vi "Get Package Dependencies from BuildSpec.vi"(0 "Path":path=path "C:/validation/Validation Framework/VI Packages/Build Specification/Validation Class/CLIVE.vipb", 11 "error in (no error)":errorcluster) -> (6 "Dependencies":string[](array[string])=["cirrus_ins_driver_silicon_delta >=2.0.0.1", "cirrus_ins_drivers_agilent_3631a >=2.0.0.1", "cirrus_ins_drivers_digital_interface >=2.1.0.1", "cirrus_ins_drivers_dmm_class >=2.0.0.1", "cirrus_ins_drivers_instek_psmx >=2.0.0.1", "cirrus_ins_drivers_ni_dc_power >=2.0.0.1", "cirrus_ins_drivers_ni_dmm >=2.0.0.1", "cirrus_ins_drivers_ni_scope >=2.0.0.1", "cirrus_ins_drivers_power_supply >=2.0.0.1", "cirrus_ins_drivers_tektronix_scope >=2.0.0.1", "ni_lib_amc >=3.3.1.22", "openg.org_lib_openg_toolkit >=4.0.1.9", "reusables >=1.3.0.2", "vigods_com_lib_advanced_encryption_standard_(aes) >=1.0.0.12"], 15 "error out":errorcluster)   [LabVIEW 2017, in "CL_G3_VIPMUtilities.lvlib"]
uses:
  CL_G3_VIPMUtilities.lvlib
  <vilib>/xml/Close Reference(Node).vi
  <vilib>/xml/Close Reference(NdList).vi
  <resource>/objmgr/DOMUserDefRef.rc
  <vilib>/xml/NI_XML.lvlib
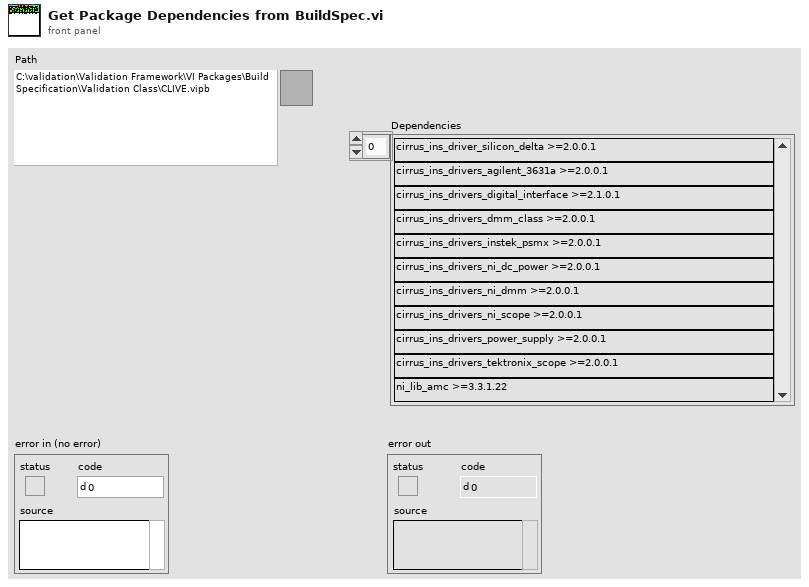
[diagram p1: front panel]
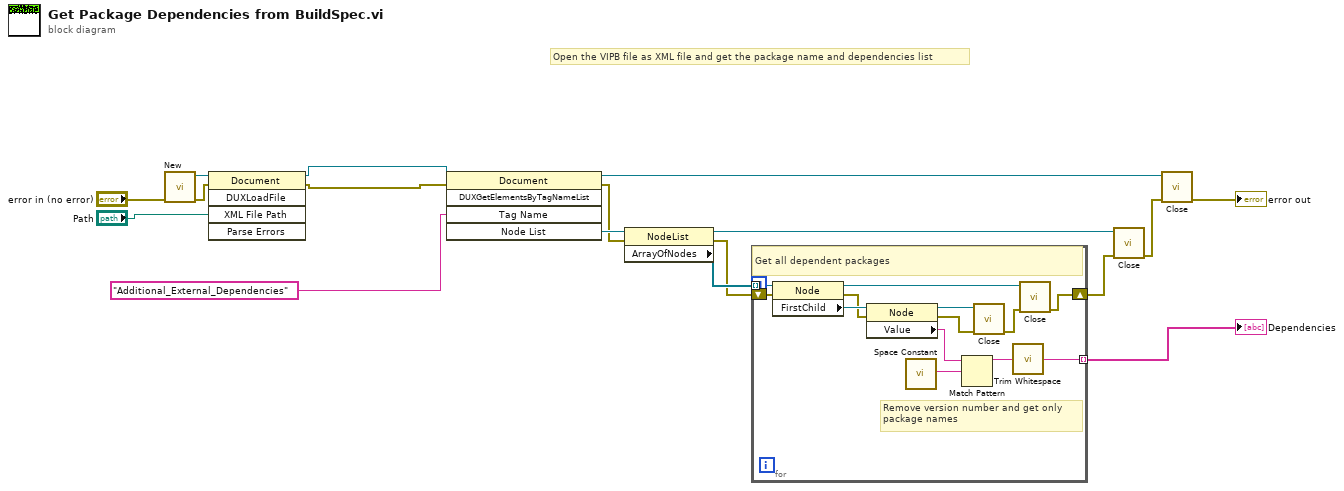
[diagram p0: block diagram]
diagram:
  # "Open the VIPB file as XML file and get the package name and dependencies list"
  n1 = call <vilib>:"New.vi"("error in (no error)"="error in (no error)") -> ("error out"=w16:errorcluster, "DOM document out"=w17:refnum<k20>)  [unwired: 7 in]
  n2 = invoke class="Document" method="DUXLoadFile"(reference=w17, error in=w16, "XML File Path"="Path") -> (reference out=w2:refnum<k20>, error out=w1:errorcluster)  [unwired: 2 in, 3 out]
  n3 = invoke class="Document" method="DUXGetElementsByTagNameList"(reference=w2, error in=w1, "Tag Name"="Additional_External_Dependencies") -> (reference out=w14:refnum<k20>, error out=w8:errorcluster, "Node List"=w13:refnum<k20>)  [unwired: 2 in, 2 out]
  n4 = property class="NodeList"(reference=w13, error in=w8) -> (reference out=w6:refnum<k20>, error out=w7:errorcluster, "ArrayOfNodes"=w9:refnum<k20>[])
  n5 = for {
    tunnel: [w18] -> w10 mode=indexing
    tunnel: w9 -> [w30] mode=indexing
    shift-right: [w22] -> w5
    shift-left: w7 -> [w28]
    # "Remove version number and get only\npackage names"
    # "Get all dependent packages"
    n6 = property class="Node"(reference=w30, error in=w28) -> (reference out=w24:refnum<k20>, error out=w25:errorcluster, "FirstChild"=w29:refnum<k20>)
    n7 = property class="Node"(reference=w29, error in=w25) -> (reference out=w26:refnum<k20>, error out=w27:errorcluster, "Value"=w21:string)
    n8 = call <vilib>:"Space Constant.vi"() -> ("String"=w19:string)
    n9 = Match Pattern(string=w21, regular expression=w19) -> (before substring=w20:string)  [unwired: 1 in, 3 out]
    n10 = call-poly <vilib>:"Close.vi"("error in (no error)"=w27, "node"=w26) -> ("error out"=w23:errorcluster)  [unwired: 7 in]
    n11 = call <vilib>:"Trim Whitespace.vi"("string"=w20) -> ("trimmed string"=w18:string)  [unwired: 1 in]
    n12 = call-poly <vilib>:"Close.vi"("error in (no error)"=w23, "node"=w24) -> ("error out"=w22:errorcluster)  [unwired: 7 in]
  }
  "Dependencies" <- w10
  n13 = call-poly <vilib>:"Close.vi"("error in (no error)"=w5, "node list"=w6) -> ("error out"=w11:errorcluster)  [unwired: 7 in]
  n14 = call-poly <vilib>:"Close.vi"("error in (no error)"=w11, "node"=w14) -> ("error out"=→"error out":errorcluster)  [unwired: 7 in]
